vi "algoritmo_8.vi"() -> ()   [LabVIEW 2024]
uses:
  <vilib>/Platform/TimedLoop/XDataNode/timing_clust.ctl
  <vilib>/Platform/TimedLoop/XDataNode/nitl_modes.ctl
  <vilib>/Platform/TimedLoop/XDataNode/wakeup.ctl
  <vilib>/MakerHub/LINX/Public/Peripherals/PWM/PWM Set Duty Cycle 1 Chan.vi
  <vilib>/MakerHub/LINX/Public/Utilities/Open Serial.vi
  <vilib>/MakerHub/LINX/Public/Peripherals/PWM/PWM Set Duty Cycle N Chans.vi
  <vilib>/platform/TimedLoop/XDataNode/XDataNode.xnode
  <vilib>/Platform/TimedLoop/XDataNode/XDNodeRunTimeDep.lvlib
  <vilib>/MakerHub/LINX/LMH-LINX.lvlib
  <vilib>/MakerHub/LINX/Public/Sensors/Distance/Ultrasonic/Ultrasonic.lvlib
  <vilib>/Analysis/NI_AALPro.lvlib
panel:
  in  "MODO":dbl
  in  "ESTIMACION":dbl(slide) scale=41.0..-41.0
  out "error":dbl
  out "i":dbl
  out "normal":dbl
  out "POLO B":dbl
  out "POLO A":dbl
  in  "polo b":dbl(slide) scale=0.0..20.0
  in  "polo a":dbl(slide) scale=0.0..50.0
  out "Xk":dbl[](array[numeric])
  out "PWM":dbl format="%0.2f"
  out "uk":dbl
  in  "Referencia":dbl(slide) scale=5.0..41.0
  out "ESTADO":dbl
  out "MINUTOS":dbl format="%#_2g"
  out "y_estimada":dbl
  out "error de estimacion":dbl
  out "THETA":cdb[](array[numeric])
  out "Waveform Chart":T1(graph)
  in  "stop":bool
  in  "Serial Port":refnum<visa-resource-name>="N/A"
  out "Error Out":errorcluster
  out "Y_Real":fxp<+/-,64,32>
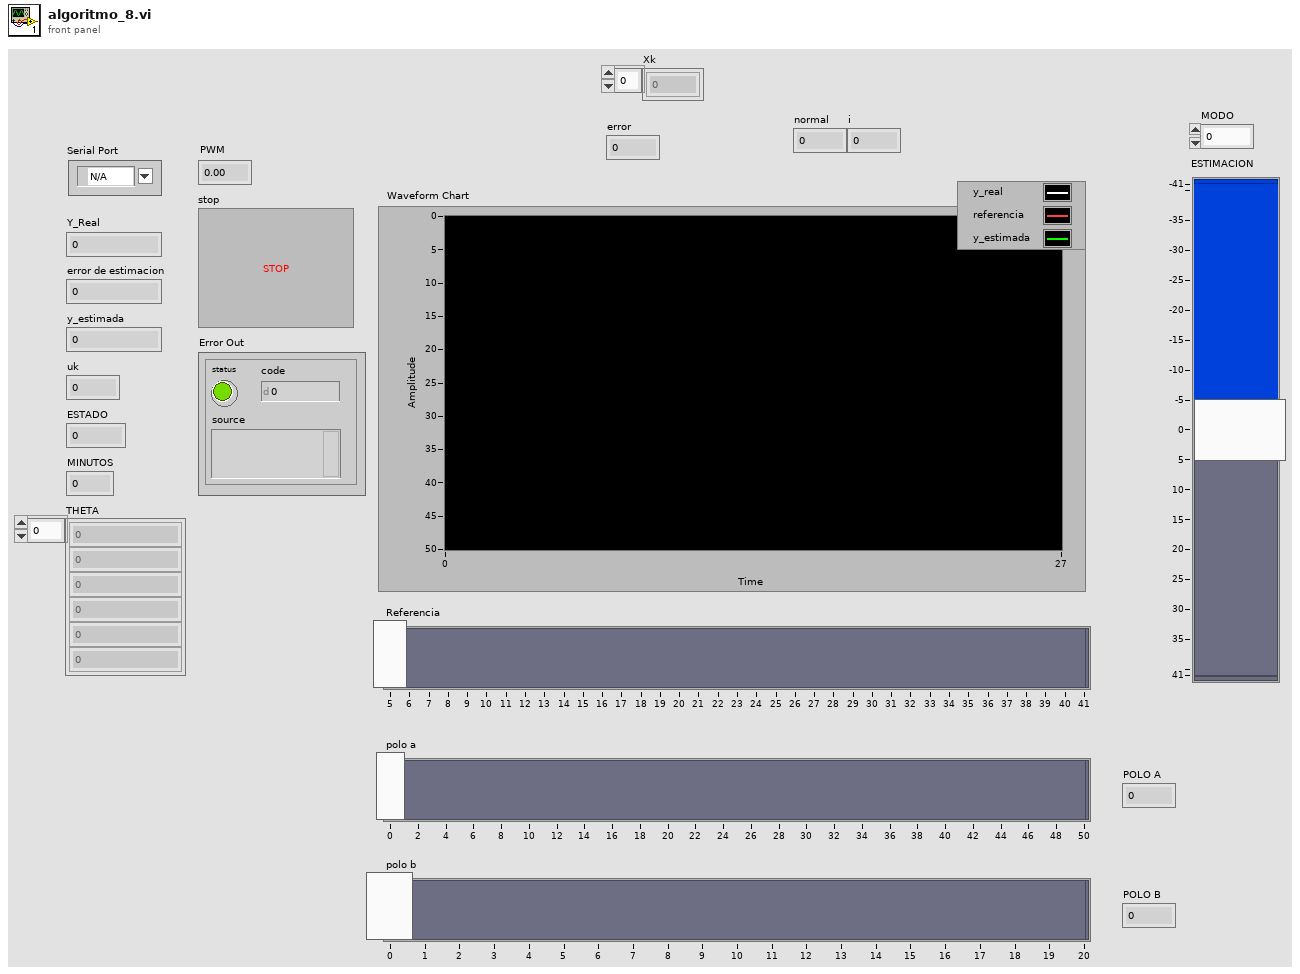
[diagram p1: front panel]
types:
  T1 = cluster{"Centimeters":dbl, "Referencia":dbl, dbl}
  T2 = typedef "LMH-LINX.lvlib/LINX Ref.ctl" = cluster{"IO":T3, "Interface":T4, "LINX Device Config":T5}
  T3 = typedef "LMH-LINX.lvlib/Platform.ctl" = enum16{"Remote", "Local"}
  T4 = typedef "LMH-LINX.lvlib/Interface.ctl" = enum16{"Serial", "TCP"}
  T5 = typedef "LMH-LINX.lvlib/Device.lvlib/LINX Device Config.ctl" = cluster{"Interface":T4, "COM Port":refnum<visa-resource-name>, "TCP Configuration":T6, "Device Family":u8, "Device ID":u8, "Device Name":string, "TCP Ref":refnum<k5>, "Channels":T7}
  T6 = typedef "LMH-LINX.lvlib/Device.lvlib/TCP Config.ctl" = cluster{"IP Address":string, "Port":u16}
  T7 = typedef "LMH-LINX.lvlib/Channels.ctl" = cluster{"DI":u8[], "DO":u8[], "AI":u8[], "AO":u8[], "PWM":u8[], "QE":u8[], "UART":u8[], "I2C 2":u8[], "SPI":u8[], "CAN":u8[], "Servo":u8[], "AI Ref (V)":dbl, "AI Resolution (Bits)":u8, "AO Ref (V)":dbl, "AO Resolution (Bits)":u8}
  T8 = typedef "XDNodeRunTimeDep.lvlib/timing_clust.ctl" = cluster{"Expected End [f-1]":u64, "Actual End [f-1]":u64, "Finished Late? [f-1]":bool, "Expected End [i-1]":u64, "Actual End [i-1]":u64, "Finished Late? [i-1]":bool, "Expected Start [i]":u64, "Actual Start [i]":u64, "Expected Start [f]":u64, "Actual Start [f]":u64, "Source Name":string, "Structure Name":string, "Period":i64, "Deadline":i64, "Offset":i64, "Start":i64, "Priority":i32, "Timeout":i32, "Mode":T9, "Wakeup Reason":T10, "Error":errorcluster, "Source Type":string, "Secondary Source Type":string, "Global End Time":u64, "Global Start Time":u64, "Frame Duration":u64, "Iteration Duration":u64, "Assigned CPU":i32, "I/O Scan Engine Mode":u32}
  T9 = typedef "XDNodeRunTimeDep.lvlib/nitl_modes.ctl" = enum32{"No Change", "Process missed periods, maintain original phase", "Discard missed periods, maintain original phase", "Process missed periods, ignore original phase", "Discard missed periods, ignore original phase"}
  T10 = typedef "XDNodeRunTimeDep.lvlib/wakeup.ctl" = enum32{"Normal", "Aborted", "Asynchronous wakeup", "Timing source error", "Timed loop error", "Timeout"}
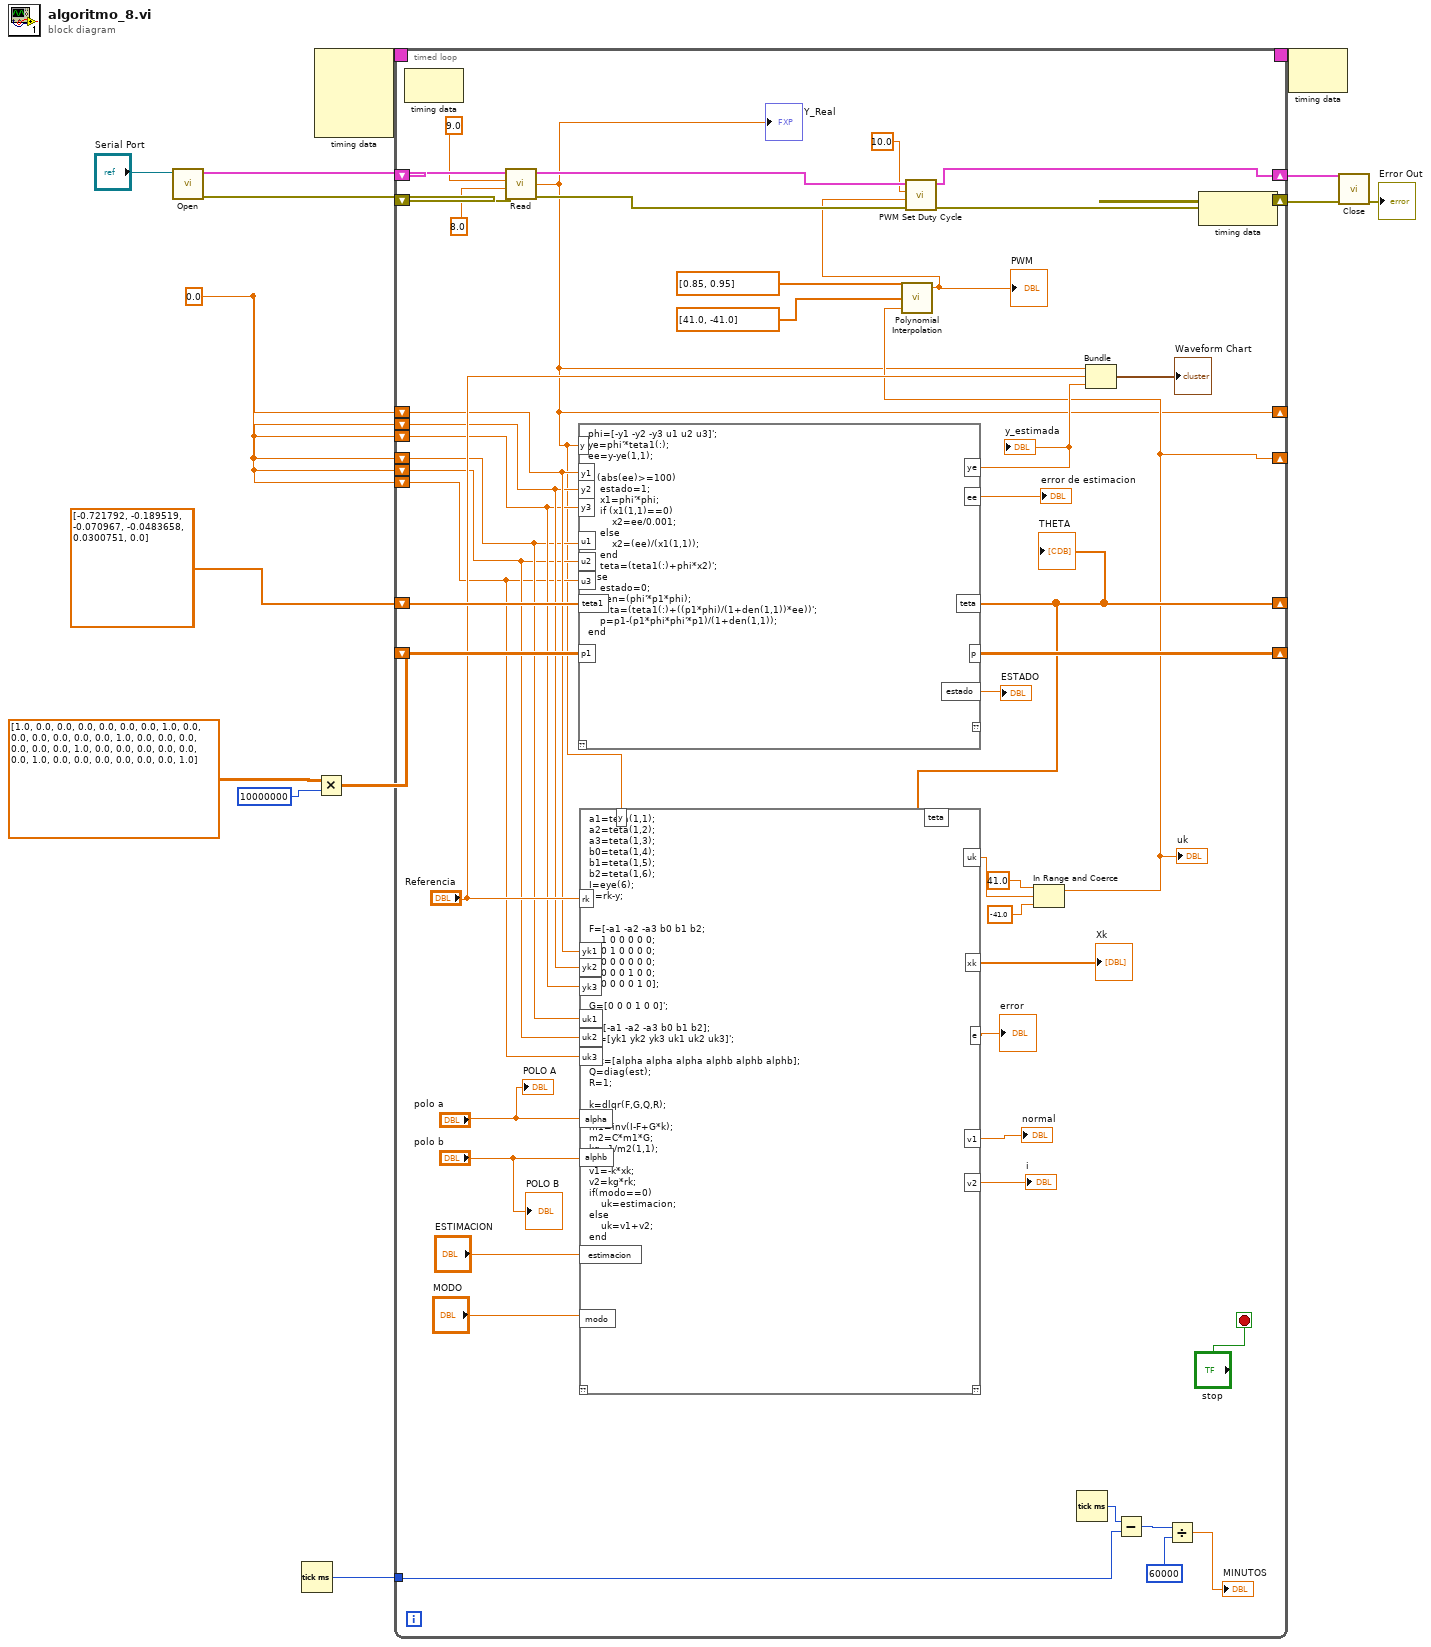
[diagram p0: block diagram]
diagram:
  (unwired) dbl[] [-0.721792, -0.189519, -0.070967, -0.0483658, 0.0300751, 0.0]
  w6 = 0.0
  n1 = call-poly <vilib>:"Open.vi"("Serial Port"="Serial Port") -> ("Error Out"=w10:errorcluster, "LINX Resource"=w12:T2)  [unwired: 8 in, 1 out]
  n2 = Tick Count (ms)() -> (millisecond timer value=w2:u32)
  n3 = node-c288() -> (w14:T8)  [unwired: 4 in]
  n4 = Multiply(x=dbl[][] [[1.0, 0.0, 0.0, 0.0, 0.0, 0.0], [0.0, 1.0, 0.0, 0.0, 0.0, 0.0], [0.0, 0.0, 1.0, 0.0, 0.0, 0.0], [0.0, 0.0, 0.0, 1.0, 0.0, 0.0], [0.0, 0.0, 0.0, 0.0, 1.0, 0.0], [0.0, 0.0, 0.0, 0.0, 0.0, 1.0]], y=10000000) -> (x*y=w3:dbl[][])
  n5 = timed-loop {
    timing: w14 -> [_]
    timing-out: [_] -> w13
    shift-right: [w48] -> w11
    shift-left: w12 -> [w60]
    shift-right: [w54] -> w9
    shift-left: w10 -> [w59]
    shift-right: [w35] -> _
    shift-left: dbl[] [-0.920929, -0.11215, 0.0219144, -0.00362395, -0.00284852, 0.0200574] -> [w47]
    shift-right: [w18] -> _
    shift-left: w6 -> [w28]
    shift-right: [w30] -> _
    shift-left: w6 -> [w25]
    shift-left: w6 -> [w27]
    shift-left: w6 -> [w26]
    shift-left: w6 -> [w24]
    shift-left: w6 -> [w23]
    shift-right: [w44] -> _
    shift-left: w3 -> [w45]
    tunnel: w2 -> [w40]
    stop <- "stop" stop-if-true
    n6 = node-c288() -> ()  [unwired: 1 in, 1 out]
    n7 = call <vilib>:"Read.vi"("Error In"=w59, "DO Channel"=8.0, "DI Channel"=9.0, "LINX Resource"=w60) -> ("Error Out"=w55:errorcluster, "Centimeters"=w18:dbl, "LINX Resource"=w56:T2)  [unwired: 4 in, 1 out]
    "Y_Real" <- w18
    n8 = script code="phi=[-y1 -y2 -y3 u1 u2 u3]';\nye=phi'*teta1(:);\nee=y-ye(1,1);\n\nif (abs(ee)>=100)\n    estado=1;\n    x1=phi'*phi;\n    if (x1(1,1)==0)\n        x2=ee/0.001;\n    else\n        x2=(ee)/(x1(1,1));\n    end\n    teta=(teta1(:)+phi*x2)';\nelse\n    estado=0;\n    den=(phi'*p1*phi);\n    teta=(teta1(:)+((p1*phi)/(1+den(1,1))*ee))';\n    p=p1-(p1*phi*phi'*p1)/(1+den(1,1));\nend"("teta1"=w47, "y1"=w28, "y2"=w27, "y3"=w26, "u1"=w25, "u2"=w24, "u3"=w23, "y"=w18, "p1"=w45) -> ("teta"=w35:dbl[], "p"=w44:dbl[][], "ye"=w43:dbl, "ee"=→"error de estimacion":dbl, "estado"=→"ESTADO":dbl)  [unwired: 1 in, 1 out]
    "THETA" <- w35
    "y_estimada" <- w43
    n9 = script code="a1=teta(1,1);\na2=teta(1,2);\na3=teta(1,3);\nb0=teta(1,4);\nb1=teta(1,5);\nb2=teta(1,6);\nI=eye(6);\ne=rk-y;\n\n\nF=[-a1 -a2 -a3 b0 b1 b2;\n    1 0 0 0 0 0;\n    0 1 0 0 0 0;\n    0 0 0 0 0 0;\n    0 0 0 1 0 0;\n    0 0 0 0 1 0];\n\nG=[0 0 0 1 0 0]';\n\nC=[-a1 -a2 -a3 b0 b1 b2];\nxk=[yk1 yk2 yk3 uk1 uk2 uk3]';\n\nest=[alpha alpha alpha alphb alphb alphb];\nQ=diag(est);\nR=1;\n\nk=dlqr(F,G,Q,R);\n\nm1=inv(I-F+G*k);\nm2=C*m1*G;\nkg=1/m2(1,1);\n\nv1=-k*xk;\nv2=kg*rk;\nif(modo==0)\n    uk=estimacion;\nelse\n    uk=v1+v2;\nend"("teta"=w35, "rk"="Referencia", "yk1"=w28, "yk2"=w27, "yk3"=w26, "uk1"=w25, "uk2"=w24, "uk3"=w23, "alpha"="polo a", "alphb"="polo b", "y"=w18, "estimacion"="ESTIMACION", "modo"="MODO") -> ("xk"=→"Xk":dbl[], "uk"=w31:dbl, "v1"=→"normal":dbl, "v2"=→"i":dbl, "e"=→"error":dbl)  [unwired: 1 in, 1 out]
    n10 = In Range and Coerce(upper limit=41.0, x=w31, lower limit=-41.0) -> (coerced(x)=w30:dbl)  [unwired: 1 out]
    "uk" <- w30
    n11 = call <vilib>:"Polynomial Interpolation.vi"("x value"=w30, "X"=dbl[] [41.0, -41.0], "Y"=dbl[] [0.85, 0.95]) -> ("interpolation value"=w50:dbl)  [unwired: 2 out]
    "PWM" <- w50
    n12 = call-poly <vilib>:"PWM Set Duty Cycle.vi"("Error In"=w55, "Duty Cycle (0-1)"=w50, "PWM Channel"=10.0, "LINX Resource"=w56) -> ("Error Out"=w54:errorcluster, "LINX Resource"=w48:T2)  [unwired: 6 in]
    n13 = Tick Count (ms)() -> (millisecond timer value=w41:u32)
    n14 = Bundle("Centimeters"=w18, "Referencia"="Referencia", w43) -> (→"Waveform Chart":T1)  [unwired: 1 in]
    n15 = Subtract(x=w41, y=w40) -> (x-y=w38:u32)
    n16 = Divide(x=w38, y=u32 60000) -> (x/y=→"MINUTOS":dbl)
    n17 = node-c288() -> ()  [unwired: 1 in, 1 out]
    "POLO A" <- "polo a"
    "POLO B" <- "polo b"
  }
  n18 = node-c288(w13) -> ()  [unwired: 1 out]
  n19 = call <vilib>:"Close.vi"("Error In"=w9, "LINX Resource"=w11) -> ("Error Out"=→"Error Out":errorcluster)  [unwired: 9 in]
